vi "Add Default Enum.vi"(6 "Hdr Name":T1, 8 "error in (no error)":errorcluster, 9 "Enum Values":u16[](array[numeric]), 11 "Tachometer in":refnum<class "Tachometer.lvclass">) -> (0 "error out":errorcluster, 3 "Tachometer out":refnum<class "Tachometer.lvclass">)   [LabVIEW 2012, in "Measurement Channels.lvlib" / "Tachometer.lvclass"]
uses:
  Tachometer.lvclass
  Common/Controls/HeaderNames.ctl
  Class Frequency/Frequency.lvclass
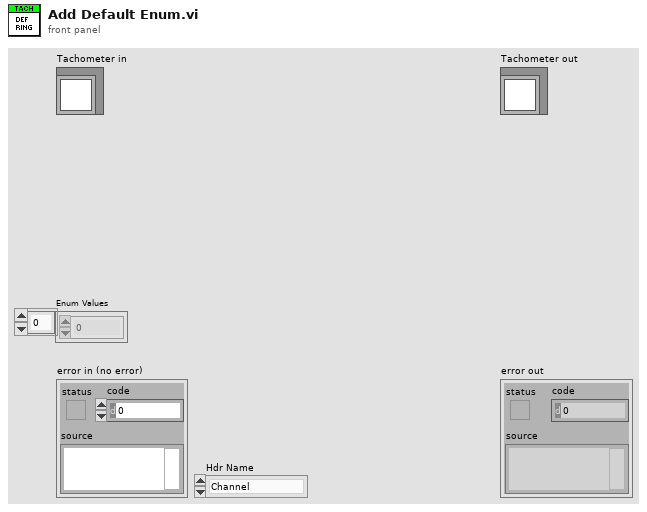
[diagram p1: front panel]
types:
  T1 = typedef "HeaderNames.ctl" = enum16{"Channel", "Device", "Spacer", "Description", "MB", "Range", "Terminal", "Coupling", "Thresh (V)", "Pulse/Rev", "Slope", "Min EU", "Min RPM", "mV/EU", "Iex", "Temp Units", "Type", "CJC Src", "CJC Val", "Ro", "Wire Cfg", "Strain Mode", "Vex", "Bridge Type", "GF", "Gauge Res", "Poisson", "Lead Res", "Init Strain", "GAF", "Scale", "Offset", "Unit (EU)", "dB?", "dB Ref", "Cal Mag", "Cal Units", "Max Temp", "Min Temp", "Max Strain", "Min Strain"}
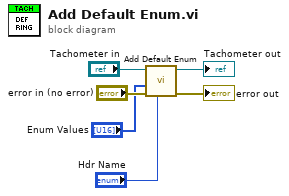
[diagram p0: block diagram]
diagram:
  n1 = call-parent "Add Default Enum.vi"("Hdr Name"="Hdr Name", "error in (no error)"="error in (no error)", "Enum Values"="Enum Values", "Frequency in"="Tachometer in") -> ("error out"=→"error out":errorcluster, "Frequency out"=→"Tachometer out":refnum<class "Tachometer.lvclass">)  [unwired: 6 in]
